vi "GE5565 DMA Interrupt Read Write Multiple MoveIn64.vi"() -> ()   [LabVIEW 2015]
uses:
  <vilib>/Platform/TimedLoop/XDataNode/timing_clust.ctl
  <vilib>/Platform/TimedLoop/XDataNode/nitl_modes.ctl
  <vilib>/Platform/TimedLoop/XDataNode/wakeup.ctl
  <vilib>/Platform/TimedLoop/XDataNode/XDataNode.xnode
  <vilib>/Platform/TimedLoop/XDataNode/XDNodeRunTimeDep.lvlib
  RefMem DMA Custom Device.lvlib
panel:
  in  "Write decimation":u32[](array[numeric])=[1, 1, 1, 1]
  in  "Read decimation":u32[](array[numeric])=[1, 1, 1, 1]
  out "Iteration Duration":i64
  out "Duration":u32
  in  "Write Enabled":bool=TRUE
  out "Numeric":i32
  in  "Data to write":dbl[][](array[numeric])=[[632.9529999919446, 1000.0580033641951, 632.9529999919446, 2.906940440898936e+231, -5.3286886514580804e+222, -2.6056933394282853e+151, -7.156383880306343e-40, -1.7467363238085046e+258, -2.4270311205663287e-175, 1.4753298638988894e-162, -1.3426130410879926e+76, 1.643060926801545e+103, -5.741333353906559e+187, 3.479924271754068e+305, 0.8412850479344235, 7.121740825496998e+190, -9.492883755239554e-94, 1.1075498683414152e+115, -1.610103260644287e+230, 1.2206393205212813e+106, -3.4489556988614912e-143, 1.6839788532006132e+308, -9.083611179879226e+226, -4.999138388987056e+252, -1.396848265976509e+153, -1.6156901514345996e-77, 5.078201317091061e+228, -7.032474044031573e+112, -3.1791549650046703e-158, 7.537090888298574e+266, -5.825269337239782e+169, -2.0675487717881096e+92], [1000.0580033641951, 632.9529999919446, 1000.0580033641951, -5.724919636444281e+259, -3.5412934410368353e+152, 1.4428981172327444e+112, -4.457727497533247e-08, 2.2688243797877682e-41, 3.8038502049438126e+286, -6.731941943127056e+307, -9.602458817991493e+229, -1.02594710746458e+152, -1.466134854835175e+225, 5.152947745650925e+230, -3.345498991233195e-80, 8.173632814654737e-194, -1.7612199822520925e-81, 1.7472151978499725e+286, -8.545632341396172e-32, 4.211405592015808e-81, 2.101064072415662e+307, 1.3426425922315837e+67, -5.190507685948668e-23, -1.335005922111333e-51, -2.2883531787919392e+229, 8.786534358092048e+189, 7.172938655978898e-25, -7.97890320094149e+102, -2.2051646463533368e+307, 2.202346326631344e+296, -3.6683837393780375e-79, 2.6567497724151404e+76], [632.9529999919446, 1000.0580033641951, -1.9887194144224296e-78, 9.417463204359133e+266, -1.1189077892199716e+297, 3.369302506338419e+307, 1.6702631324723968e-80, 4.941487405273079e+153, -1.5431812183401114e+231, 4.584407096181318e+105, -1.2628305856551255e-82, 1.5527507064618875e+144, -1.1414448856415074e+77, 4.0862304438258354e+93, -4.348942625254957e-103, 7.191670164467337e+112, -4.171680584616603e+186, -8.869860281421606e+122, 9.359555906427844e-79, 1.2454095446860644e+153, -3.3401652140694516e-34, -3.0009451382216142e+296, -8.144409909831617e+229, 1.6336253586608878e+260, -1.2361411739522516e+284, -1.7438017208894331e-155, -7.575081977324324e+199, 1.8189032773553975e+142, -2.6412286718746365e+169, 7.1596366259451545e+103, 1.926518961568148e-252, 8.814735000151876e+268], [632.9529999919446, 1000.0580033641951, 632.9529999919446, 2.906940440898936e+231, -5.3286886514580804e+222, -2.6056933394282853e+151, -7.156383880306343e-40, -1.7467363238085046e+258, -2.4270311205663287e-175, 1.4753298638988894e-162, -1.3426130410879926e+76, 1.643060926801545e+103, -5.741333353906559e+187, 3.479924271754068e+305, 0.8412850479344235, 7.121740825496998e+190, -9.492883755239554e-94, 1.1075498683414152e+115, -1.610103260644287e+230, 1.2206393205212813e+106, -3.4489556988614912e-143, 1.6839788532006132e+308, -9.083611179879226e+226, -4.999138388987056e+252, -1.396848265976509e+153, -1.6156901514345996e-77, 5.078201317091061e+228, -7.032474044031573e+112, -3.1791549650046703e-158, 7.537090888298574e+266, -5.825269337239782e+169, -2.0675487717881096e+92]]
  in  "Channel offset write in channels":u32[](array[numeric])=[3, 35, 102, 1000]
  in  "Channel count write":u32[](array[numeric])=[32, 32, 32, 32]
  in  "Channel offset read in channels":u32[](array[numeric])=[0, 32, 100, 1000]
  in  "Channel count read":u32[](array[numeric])=[32, 32, 32, 32]
  out "Data":dbl[][](array[numeric])
  in  "stop":bool
  # "Note: This VI requires the GE5565PIORC_NetworkInterrupts_DMA.inf\ndevice driver."
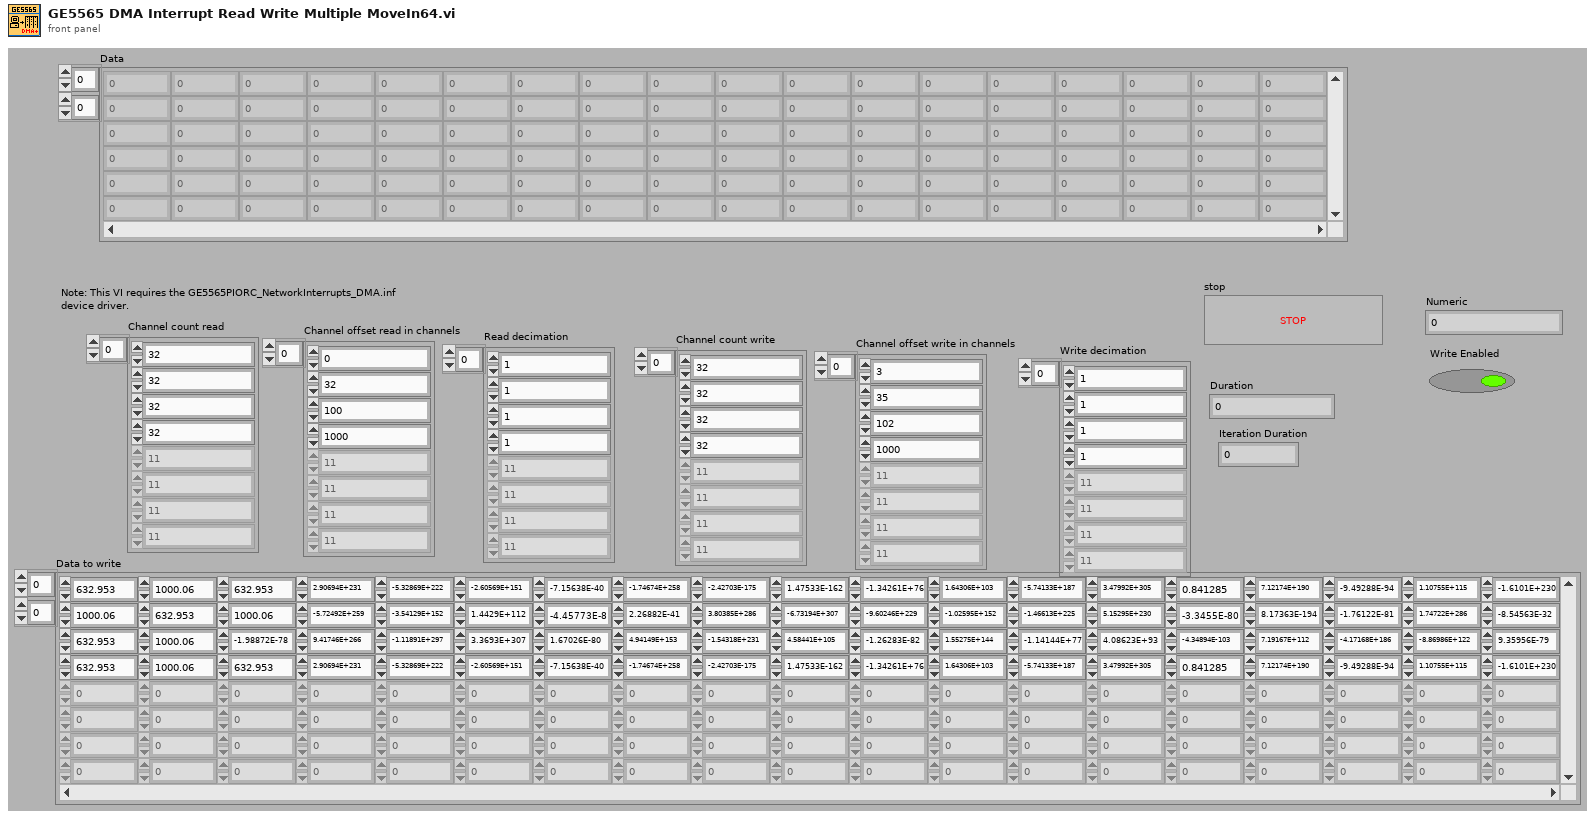
[diagram p1: front panel]
types:
  T1 = cluster{"VMIC 5565 Resource":refnum<visa-resource-name>, "MEMACC Resource":refnum<visa-resource-name>, "byte count":u32, "mem offset":u32}
  T2 = typedef "XDNodeRunTimeDep.lvlib/timing_clust.ctl" = cluster{"Expected End [f-1]":u64, "Actual End [f-1]":u64, "Finished Late? [f-1]":bool, "Expected End [i-1]":u64, "Actual End [i-1]":u64, "Finished Late? [i-1]":bool, "Expected Start [i]":u64, "Actual Start [i]":u64, "Expected Start [f]":u64, "Actual Start [f]":u64, "Source Name":string, "Structure Name":string, "Period":i64, "Deadline":i64, "Offset":i64, "Start":i64, "Priority":i32, "Timeout":i32, "Mode":T3, "Wakeup Reason":T4, "Error":errorcluster, "Source Type":string, "Secondary Source Type":string, "Global End Time":u64, "Global Start Time":u64, "Frame Duration":u64, "Iteration Duration":u64, "Assigned CPU":i32, "I/O Scan Engine Mode":u32}
  T3 = typedef "XDNodeRunTimeDep.lvlib/nitl_modes.ctl" = enum32{"No Change", "Process missed periods, maintain original phase", "Discard missed periods, maintain original phase", "Process missed periods, ignore original phase", "Discard missed periods, ignore original phase"}
  T4 = typedef "XDNodeRunTimeDep.lvlib/wakeup.ctl" = enum32{"Normal", "Aborted", "Asynchronous wakeup", "Timing source error", "Timed loop error", "Timeout"}
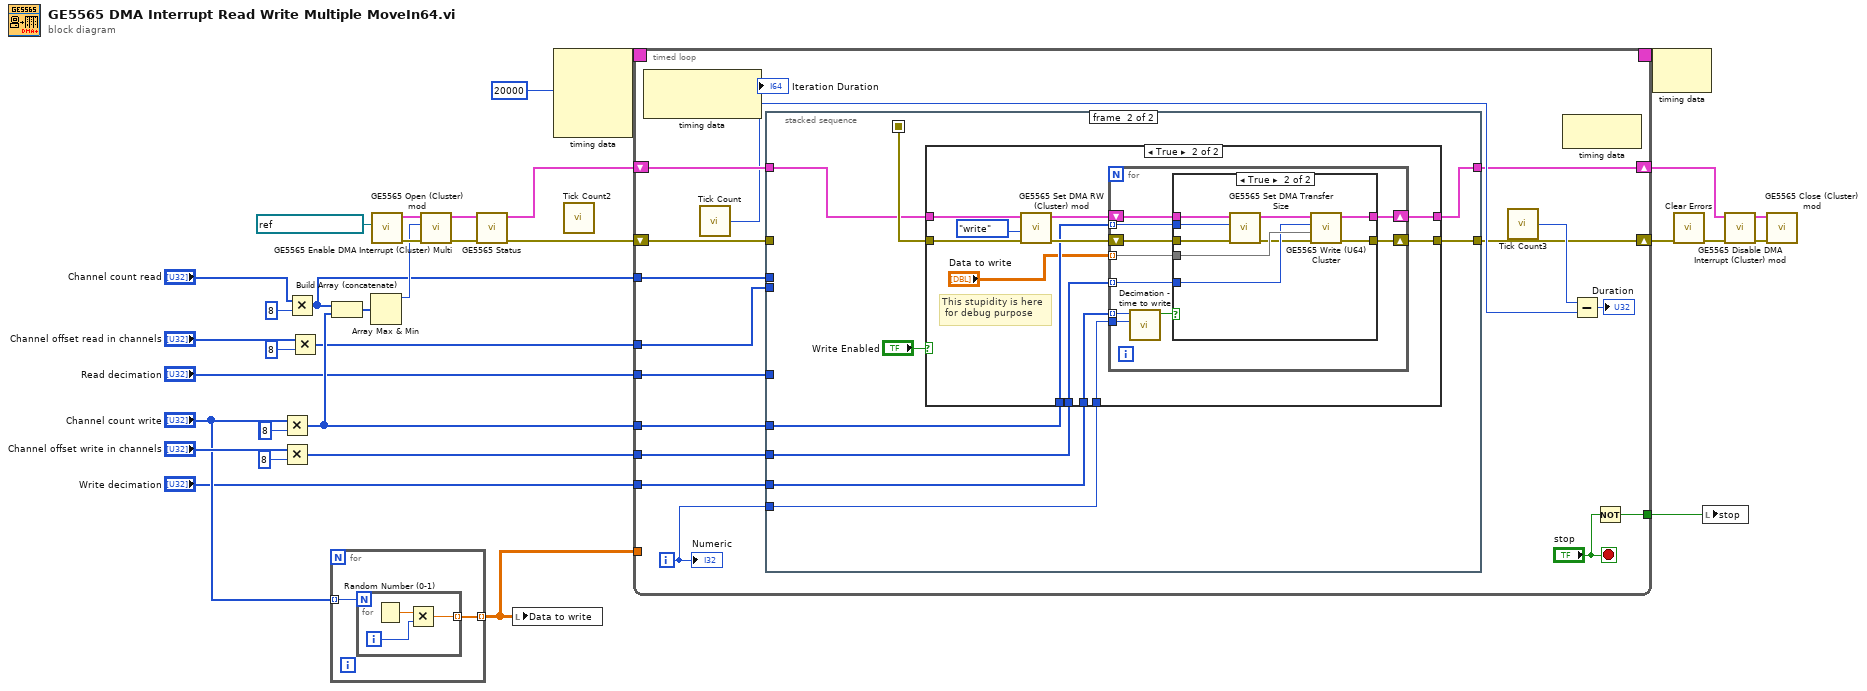
[diagram p0: block diagram]
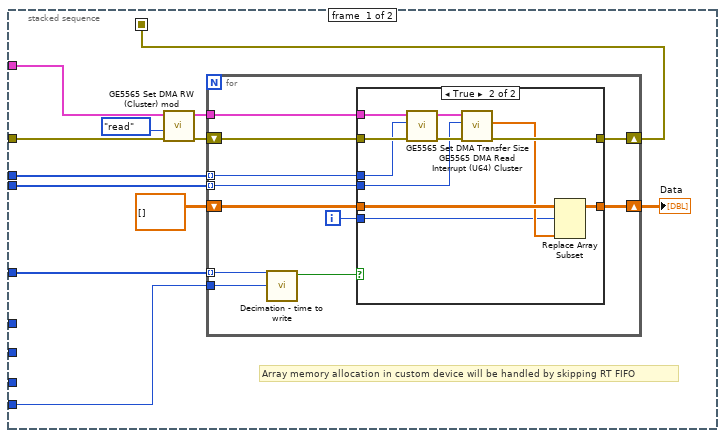
[diagram p2: hidden frame]
diagram:
  (unwired) u32 8 ("y")
  n1 = Multiply(x="Channel count write", y=u32 8) -> (x*y=w8:u32[])
  n2 = Multiply(x="Channel offset write in channels", y=u32 8) -> (x*y=w14:u32[])
  n3 = Multiply(x="Channel count read", y=u32 8) -> (x*y=w2:u32[])
  n4 = Multiply(x="Channel offset read in channels", y=u32 8) -> (x*y=w1:u32[])
  n5 = for {
    tunnel: "Channel count write" -> [w35] mode=indexing
    tunnel: [w34] -> w10 mode=indexing
    n6 = for {
      N: w35 -> [_]
      tunnel: [w37] -> w34 mode=indexing
      i -> [w36]
      n7 = Random Number (0-1)() -> (number: 0 to 1=w38:dbl)
      n8 = Multiply(x=w38, y=w36) -> (x*y=w37:dbl)
    }
  }
  n9 = Build Array (concatenate)(w2, w8) -> (w9:u32[])
  n10 = Array Max & Min(array=w9) -> (max value=w19:u32)  [unwired: 3 out]
  n11 = call "GE5565 Open (Cluster) mod.vi"("VISA resource name (empty)"=refnum<visa-resource-name> "PXI4::12::INSTR") -> ("error out"=w29:errorcluster, "VMIC-5565"=w27:T1)  [unwired: 5 in]
  n12 = call "GE5565 Enable DMA Interrupt (Cluster) Multi.vi"("error in (no error)"=w29, "transfer size (1024 bytes)"=w19, "VMIC reference in"=w27) -> ("error out"=w7:errorcluster, "VMIC reference out"=w6:T1)  [unwired: 3 in]
  n13 = call "GE5565 Status.vi"("error in (no error)"=w7, "VMIC reference in"=w6) -> ("error out"=w11:errorcluster, "VMIC reference out"=w5:T1)  [unwired: 3 in, 1 out]
  n14 = local write "Data to write"(w10) -> ()
  n15 = node-c288(i64 20000 ("Period")) -> (w33:T2)  [unwired: 3 in]
  n16 = call "Tick Count2"() -> ()  [unwired: 1 out]
  n17 = timed-loop {
    timing: w33 -> [_]
    timing-out: [_] -> w32
    shift-right: [w45] -> w23
    shift-left: w11 -> [w51]
    tunnel: [w54] -> w24
    tunnel: w2 -> [w50]
    tunnel: w1 -> [w49]
    shift-right: [w42] -> w25
    shift-left: w5 -> [w52]
    tunnel: w8 -> [w44]
    tunnel: w14 -> [w43]
    tunnel: w10 -> [_]
    tunnel: "Read decimation" -> [w41]
    tunnel: "Write decimation" -> [w40]
    i -> [w39]
    stop <- "stop" stop-if-true
    n18 = node-c288() -> (→"Iteration Duration":i64)  [unwired: 1 in, 1 out]
    n19 = call "Tick Count"() -> ("Tick Count(uSec)"=w46:u32)
    n20 = stacked-sequence {
      seq-local: [w62 _] -> [_ w100]
      tunnel: w52 -> [w64 w99]
      tunnel: w51 -> [w65 _]
      tunnel: w50 -> [w61 _]
      tunnel: w49 -> [w60 _]
      tunnel: [_ w98] -> w45
      tunnel: w44 -> [_ w96]
      tunnel: w43 -> [_ w95]
      tunnel: [_ w94] -> w42
      tunnel: w41 -> [w56 _]
      tunnel: w40 -> [_ w93]
      tunnel: w39 -> [w57 w92]
      frame #0 {
        # "Array memory allocation in custom device will be handled by skipping RT FIFO"
        n21 = call "GE5565 Set DMA RW (Cluster) mod.vi"("error in (no error)"=w65, "operation (read)"=enum16{"read", "write"}."read", "VMIC-5565"=w64) -> ("error out"=w67:errorcluster, "VMIC-5565"=w63:T1)  [unwired: 3 in]
        n22 = for {
          shift-right: [w78] -> w62
          shift-left: w67 -> [w76]
          tunnel: w61 -> [w75] mode=indexing
          tunnel: w60 -> [w74] mode=indexing
          tunnel: w63 -> [w73]
          shift-right: [w77] -> w58
          shift-left: dbl[][] [] ("Data") -> [w72]
          tunnel: w57 -> [w69]
          tunnel: w56 -> [w70] mode=indexing
          i -> [w71]
          n23 = call "Decimation - time to write.vi"("Iteration"=w69, "Decimation"=w70) -> ("Ready"=w68:bool)  [unwired: 9 in]
          n24 = case shown="True" w68 {
            tunnel: [w79 w91] -> w78
            tunnel: [w80 w84] -> w77
            tunnel: w76 -> [w79 w90]
            tunnel: w75 -> [_ w87]
            tunnel: w74 -> [_ w86]
            tunnel: w73 -> [_ w85]
            tunnel: w72 -> [w80 w83]
            tunnel: w71 -> [_ w81]
            frame False {
            }
            frame True {
              n25 = call "GE5565 Set DMA Transfer Size.vi"("error in (no error)"=w90, "Transfer Size"=w87, "VMIC-5565"=w85) -> ("error out"=w89:errorcluster, "VMIC-5565"=w88:T1)  [unwired: 3 in]
              n26 = call "GE5565 DMA Read Interrupt (U64) Cluster.vi"("error in (no error)"=w89, "RM offset (0)"=w86, "VMIC reference in"=w88) -> ("error out"=w91:errorcluster, "buffer"=w82:dbl[])  [unwired: 6 in, 1 out]
              n27 = Replace Array Subset(array=w83, new element=w82, index (row)=w81) -> (w84:dbl[][])  [unwired: 1 in]
            }
          }
        }
        "Data" <- w58
      }
      frame #1 {
        n28 = case shown="True" "Write Enabled" {
          tunnel: w99 -> [w102 w114]
          tunnel: w100 -> [w101 w113]
          tunnel: [w101 w111] -> w98
          tunnel: [w102 w110] -> w94
          tunnel: w96 -> [_ w108]
          tunnel: w95 -> [_ w107]
          tunnel: w93 -> [_ w104]
          tunnel: w92 -> [_ w103]
          frame False {
          }
          frame True {
            # "This stupidity is here\n for debug purpose"
            n29 = call "GE5565 Set DMA RW (Cluster) mod.vi"("error in (no error)"=w113, "operation (read)"=enum16{"read", "write"}."write", "VMIC-5565"=w114) -> ("error out"=w112:errorcluster, "VMIC-5565"=w109:T1)  [unwired: 3 in]
            n30 = for {
              shift-right: [w124] -> w111
              shift-left: w112 -> [w122]
              shift-right: [w123] -> w110
              shift-left: w109 -> [w121]
              tunnel: w108 -> [w120] mode=indexing
              tunnel: w107 -> [w118] mode=indexing
              tunnel: "Data to write" -> [w119] mode=indexing
              tunnel: w104 -> [w116] mode=indexing
              tunnel: w103 -> [w115]
              n31 = call "Decimation - time to write.vi"("Iteration"=w115, "Decimation"=w116) -> ("Ready"=w117:bool)  [unwired: 9 in]
              n32 = case shown="True" w117 {
                tunnel: [w125 w135] -> w124
                tunnel: [w126 w134] -> w123
                tunnel: w122 -> [w125 w133]
                tunnel: w121 -> [w126 w132]
                tunnel: w120 -> [_ w131]
                tunnel: w119 -> [_ w130]
                tunnel: w118 -> [_ w129]
                frame False {
                }
                frame True {
                  n33 = call "GE5565 Set DMA Transfer Size.vi"("error in (no error)"=w133, "Transfer Size"=w131, "VMIC-5565"=w132) -> ("error out"=w127:errorcluster, "VMIC-5565"=w128:T1)  [unwired: 3 in]
                  n34 = call "GE5565 Write (U64) Cluster.vi"("error in (no error)"=w127, "buffer"=w130, "offset (0)"=w129, "VMIC reference in"=w128) -> ("error out"=w135:errorcluster, "VMIC reference out"=w134:T1)  [unwired: 6 in]
                }
              }
            }
          }
        }
      }
    }
    n35 = call "Tick Count3"() -> ("Tick Count(uSec)"=w48:u32)
    n36 = node-c288() -> ()  [unwired: 1 in, 1 out]
    n37 = Subtract(x=w48, y=w46) -> (x-y=→"Duration":u32)
    n38 = Not(x="stop") -> (.not. x?=w54:bool)
    "Numeric" <- w39
  }
  n39 = node-c288(w32) -> ()  [unwired: 1 out]
  n40 = call <vilib>:"Clear Errors.vi"("error in (no error)"=w23) -> ("error out"=w22:errorcluster)  [unwired: 5 in, 1 out]
  n41 = local write "stop"(w24) -> ()
  n42 = call "GE5565 Disable DMA Interrupt (Cluster) mod.vi"("error in (no error)"=w22, "VMIC reference in"=w25) -> ("error out"=w28:errorcluster, "VMIC reference out"=w26:T1)  [unwired: 4 in]
  n43 = call "GE5565 Close (Cluster) mod.vi"("error in (no error)"=w28, "VMIC reference in"=w26) -> ()  [unwired: 5 in, 1 out]
